vi "Save data waveform or image.vi"(0 "Autosave Folder":path, 5 "Scan Folder":path, 7 "Image Data":T1, 9 "Numeric Data":dbl[](array[numeric]), 11 "Data Format":enum16{"Image", "Numeric Data"}(ring)) -> ()   [LabVIEW 2013, in "GeneralDevice.lvclass"]
uses:
  GeneralDevice.lvclass
  <vilib>/vision/Image Controls.llb/IMAQ Image.ctl
panel:
  in  "Write period (s)":dbl=10.0 caption="Time Target (s)"
  out "image::1":T1(plugin-control) caption="HPD_CCD"
  out "Writing to file!":bool
  in  "stop":bool
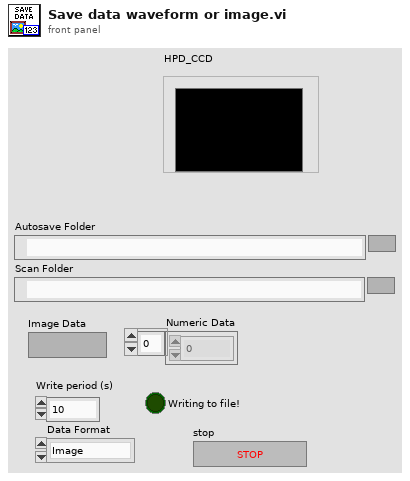
[diagram p1: front panel]
types:
  T1 = typedef "IMAQ Image.ctl" = refnum<image>
  T2 = enum16{"open", "replace", "create", "open or create", "replace or create", "replace or create with confirmation"}
  T3 = typedef "Image Type" = u32
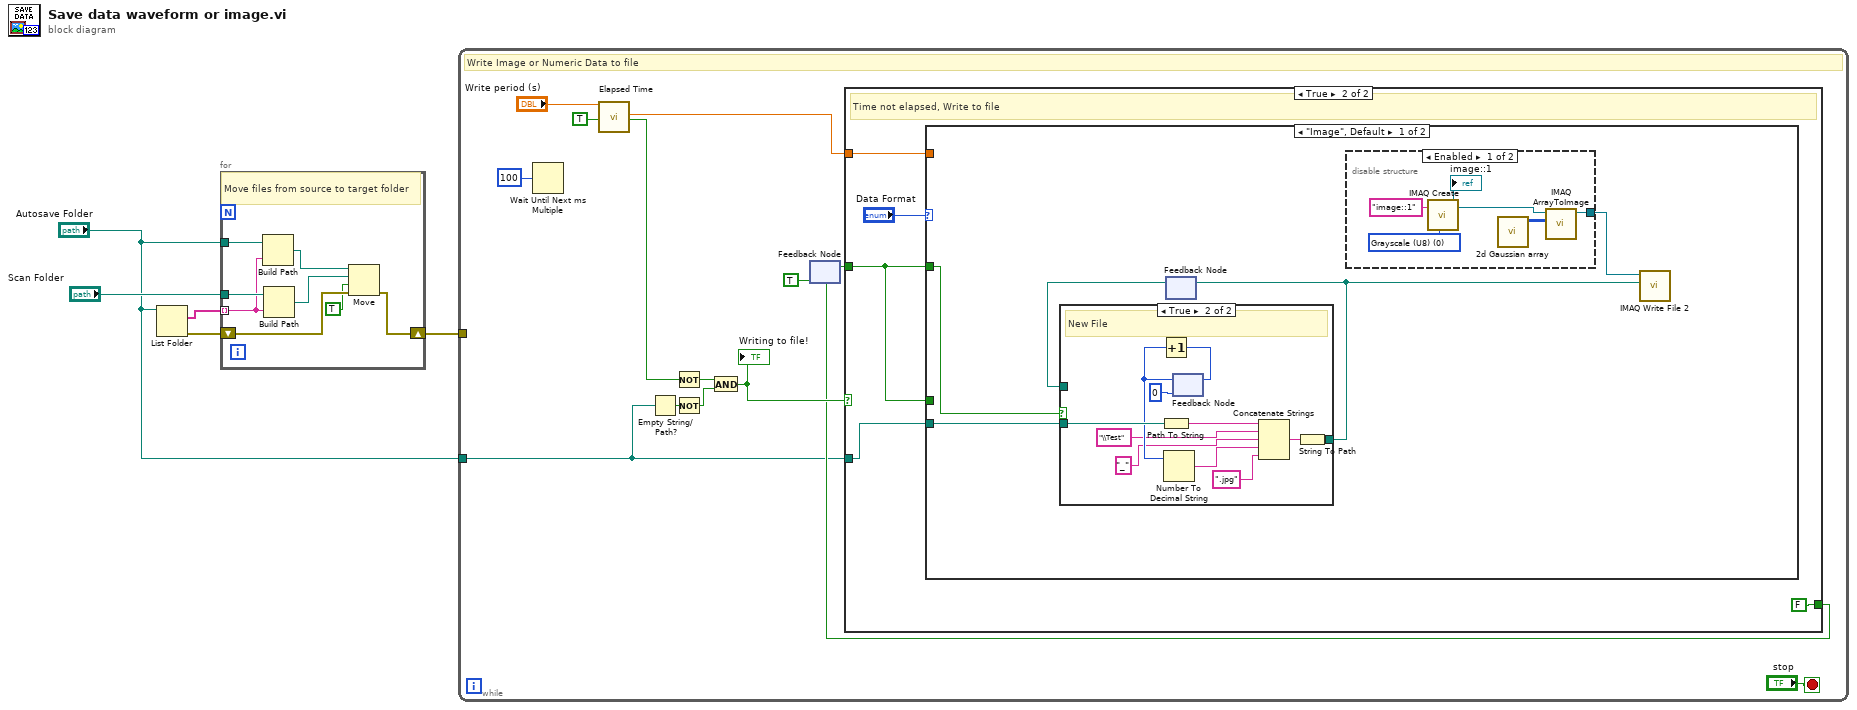
[diagram p0: block diagram]
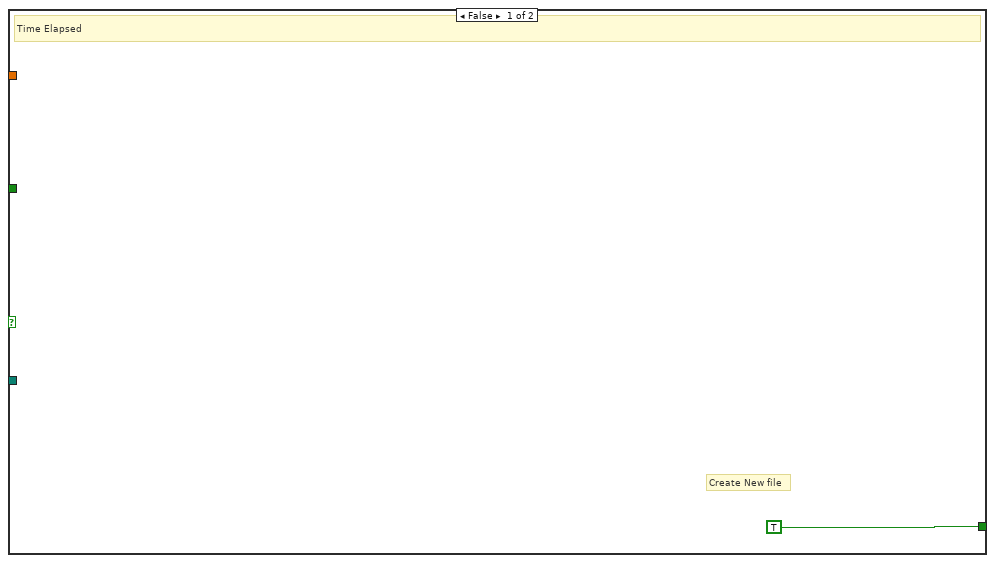
[diagram p2: hidden frame]
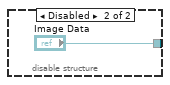
[diagram p3: hidden frame]
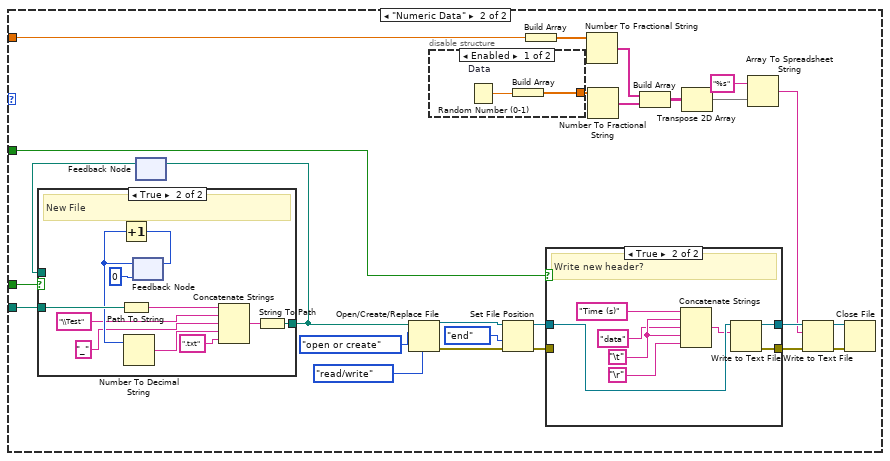
[diagram p5: hidden frame]
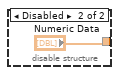
[diagram p6: hidden frame]
diagram:
  n1 = List Folder(path="Autosave Folder") -> (filenames=w4:string[], error out=w3:errorcluster)  [unwired: 3 in, 2 out]
  n2 = for {
    tunnel: "Autosave Folder" -> [w13]
    tunnel: "Scan Folder" -> [w12]
    tunnel: w4 -> [w11] mode=indexing
    shift-right: [w7] -> w2
    shift-left: w3 -> [w8]
    # "Move files from source to target folder"
    n3 = Build Path(base path=w13, name or relative path=w11) -> (appended path=w10:path)
    n4 = Build Path(base path=w12, name or relative path=w11) -> (appended path=w9:path)
    n5 = Move(source path=w10, error in=w8, 9:TRUE ("overwrite (F)"), 10:w9) -> (error out=w7:errorcluster)  [unwired: 1 in, 2 out]
  }
  n6 = while {
    tunnel: w2 -> [_]
    tunnel: "Autosave Folder" -> [w14]
    stop <- "stop" stop-if-true
    # "Write Image or Numeric Data to file"
    n7 = Wait Until Next ms Multiple(millisecond multiple=u32 100) -> ()  [unwired: 1 out]
    n8 = call "Elapsed Time"("Time Target (s)"="Write period (s)", "Auto Reset"=TRUE) -> ("Elapsed Time (s)"=w16:dbl, "Time has Elapsed"=w15:bool)  [unwired: 10 in, 6 out]
    n9 = Empty String/Path?(string/path=w14) -> (empty?=w25:bool)
    n10 = Not(x=w15) -> (.not. x?=w24:bool)
    n11 = Not(x=w25) -> (.not. x?=w23:bool)
    n12 = And(x=w24, y=w23) -> (x .and. y?=w22:bool)
    "Writing to file!" <- w22
    n13 = feedback #1(TRUE) -> (w18:bool)
    n14 = case shown="True" w22 {
      tunnel: w14 -> [_ w30]
      tunnel: w16 -> [_ w33]
      tunnel: [TRUE FALSE] -> w19
      tunnel: w18 -> [_ w29]
      frame False {
        # "Create New file"
        # "Time Elapsed"
      }
      frame True {
        # "Time not elapsed, Write to file"
        n15 = case shown="\"Image\", Default" "Data Format" {
          tunnel: w33 -> [_ w64]
          tunnel: w29 -> [w34 w61]
          tunnel: w29 -> [_ w59]
          tunnel: w30 -> [w38 w58]
          frame "Image", Default {
            n16 = feedback #2() -> (w35:path)  [unwired: 1 in]
            n17 = case shown="True" w34 {
              tunnel: w38 -> [_ w56]
              tunnel: [w45 w46] -> w36
              tunnel: w35 -> [w45 _]
              frame False {
                # "Write To same File"
              }
              frame True {
                # "New File"
                n18 = Path To String(path=w56) -> (string=w47:string)
                n19 = feedback #3(0) -> (w51:i32)
                n20 = Increment(x=w51) -> (x+1=w52:i32)
                n21 = Number To Decimal String(number=w51) -> (decimal integer string=w53:string)  [unwired: 1 in]
                n22 = feedback-in #3(w52) -> ()
                n23 = Concatenate Strings(w47, "\\Test" ("string"), "_" ("string"), w53, ".jpg" ("string")) -> (w55:string)
                n24 = String To Path(string=w55) -> (path=w46:path)
              }
            }
            n25 = feedback-in #2(w36) -> ()
            n26 = disable-structure shown="Enabled" {
              disable-tunnel: [w42 "Image Data"] -> w37
              frame Enabled {
                w41 = T3 0 items=["Grayscale (U8)", "Grayscale (I16)", "Grayscale (SGL)", "Complex (CSG)", "RGB (U32)", "HSL (U32)", "RGB (U64)", "Grayscale (U16)"] ("Image Type")
                n27 = call "IMAQ Create"("Image Name"="image::1", "Image Type"=w41) -> ("New Image"=w39:T1)  [unwired: 3 in, 1 out]
                "image::1" <- w39
                n28 = call "2d Gaussian array.vi"() -> ("Array"=w43:u8[][])  [unwired: 11 in]
                n29 = call "IMAQ ArrayToImage"("Image Pixels (U8)"=w43, "Image"=w39) -> ("Image Out"=w42:T1)  [unwired: 8 in, 1 out]
              }
              frame Disabled {
              }
            }
            n30 = call-poly "IMAQ Write File 2"("File Path"=w36, "Image"=w37) -> ()  [unwired: 8 in, 2 out]
          }
          frame "Numeric Data" {
            n31 = feedback #4() -> (w60:path)  [unwired: 1 in]
            n32 = case shown="True" w59 {
              tunnel: w58 -> [_ w95]
              tunnel: [w85 w94] -> w57
              tunnel: w60 -> [w85 _]
              frame False {
                # "Write To same File"
              }
              frame True {
                # "New File"
                n33 = Path To String(path=w95) -> (string=w86:string)
                n34 = feedback #5(0) -> (w90:i32)
                n35 = Increment(x=w90) -> (x+1=w91:i32)
                n36 = Number To Decimal String(number=w90) -> (decimal integer string=w92:string)  [unwired: 1 in]
                n37 = feedback-in #5(w91) -> ()
                n38 = Concatenate Strings(w86, "\\Test" ("string"), "_" ("string"), w92, ".txt" ("string")) -> (w96:string)
                n39 = String To Path(string=w96) -> (path=w94:path)
              }
            }
            n40 = feedback-in #4(w57) -> ()
            n41 = Open/Create/Replace File(file path (use dialog)=w57, operation (0:open)=T2."open or create", access (0:read/write)=enum16{"read/write", "read-only", "write-only"}."read/write") -> (refnum out=w74:refnum<file>, error out=w75:errorcluster)  [unwired: 3 in, 1 out]
            n42 = disable-structure shown="Enabled" {
              disable-tunnel: [w82 "Numeric Data"] -> w62
              frame Enabled {
                n43 = Random Number (0-1) "Data"() -> (number: 0 to 1=w83:dbl)
                n44 = Build Array(w83) -> (w82:dbl[])
              }
              frame Disabled {
              }
            }
            n45 = Set File Position(refnum=w74, from (0:start)=enum16{"start", "end", "current"}."end", error in=w75) -> (refnum out=w72:refnum<file>, error out=w73:errorcluster)  [unwired: 1 in]
            n46 = Build Array(w64) -> (w63:dbl[])
            n47 = case shown="True" w61 {
              tunnel: [w97 w106] -> w77
              tunnel: [w98 w105] -> w76
              tunnel: w73 -> [w98 _]
              tunnel: w72 -> [w97 w104]
              frame False {
              }
              frame True {
                w102 = "\t"
                # "Write new header?"
                n48 = Concatenate Strings("Time (s)" ("string"), w102, "data" ("string"), w102, "\r") -> (w99:string)
                n49 = Write to Text File(file (use dialog)=w104, text=w99) -> (refnum out=w106:refnum<file>, error out=w105:errorcluster)  [unwired: 2 in, 1 out]
              }
            }
            n50 = Number To Fractional String(number=w63) -> (F-format string=w65:string[])  [unwired: 3 in]
            n51 = Number To Fractional String(number=w62) -> (F-format string=w70:string[])  [unwired: 3 in]
            n52 = Build Array(w65, w70) -> (w69:string[][])
            n53 = Transpose 2D Array(2D array=w69) -> (transposed array=w68:string[][])
            n54 = Array To Spreadsheet String(array=w68, 3:"%s" ("format string")) -> (spreadsheet string=w66:string)  [unwired: 1 in]
            n55 = Write to Text File(file (use dialog)=w77, text=w66, error in=w76) -> (refnum out=w80:refnum<file>, error out=w81:errorcluster)  [unwired: 1 in, 1 out]
            n56 = Close File(refnum=w80, error in=w81) -> ()  [unwired: 2 out]
          }
        }
      }
    }
    n57 = feedback-in #1(w19) -> ()
  }
